vi "Main.vi"(8 "error in":errorcluster, 11 "Table in":refnum<class "Table.lvclass">) -> (0 "error out":errorcluster, 3 "Table out":refnum<class "Table.lvclass">)   [LabVIEW 2023, in "Table.lvclass"]
uses:
  Table.lvclass
  C:/Program Files (x86)/National Instruments/LabVIEW 2023/vi.lib/addons/_Workers/Library/Classes/Worker/Worker.lvclass
  <vilib>/addons/_Workers/Library/Classes/Worker/Worker.lvclass/Worker.ctl
  Philosopher/Initialization Data.ctl
  <vilib>/addons/_Workers/Library/Classes/Message Queue/Message Queue.lvclass
  Hungry.ctl
  Fork.ctl
  Philosopher/Philosopher.lvclass
  Table.lvclass/Table.ctl
  d0df4b09-6abd-41e7-b449-a85035083f06.vi
  <vilib>/addons/_Workers/Library/Classes/Message/Enqueue Message to Queue.vi
  <vilib>/addons/_Workers/Library/Classes/Worker/Worker.lvclass
  <vilib>/addons/_Workers/Library/Classes/Message/Message.lvclass
  C:/Program Files (x86)/National Instruments/LabVIEW 2023/vi.lib/addons/_Workers/Library/Classes/Workers Object/Workers Object.lvclass
  C:/Projects/DPP Workers/Workers/Table/Table.lvclass
panel:
  in  "The End":bool
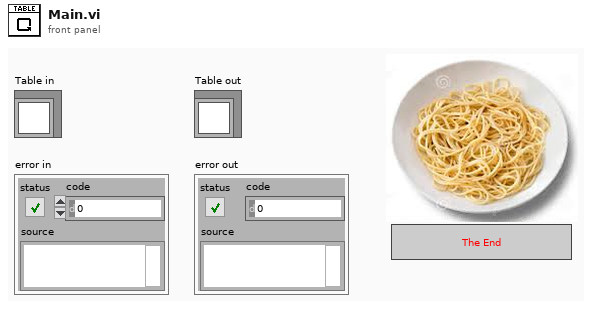
[diagram p1: front panel]
types:
  T1 = typedef "Philosopher.lvclass/Initialization Data.ctl" = cluster{"ID":i32, "MGQ Table":refnum<class "Message Queue.lvclass">}
  T2 = typedef "Table.lvclass/Hungry.ctl" = enum16{"NO", "YES"}
  T3 = typedef "Table.lvclass/Fork.ctl" = enum16{"FREE", "IN USE"}
  T4 = typedef "Workers.lvlib/Case Label.ctl" = string
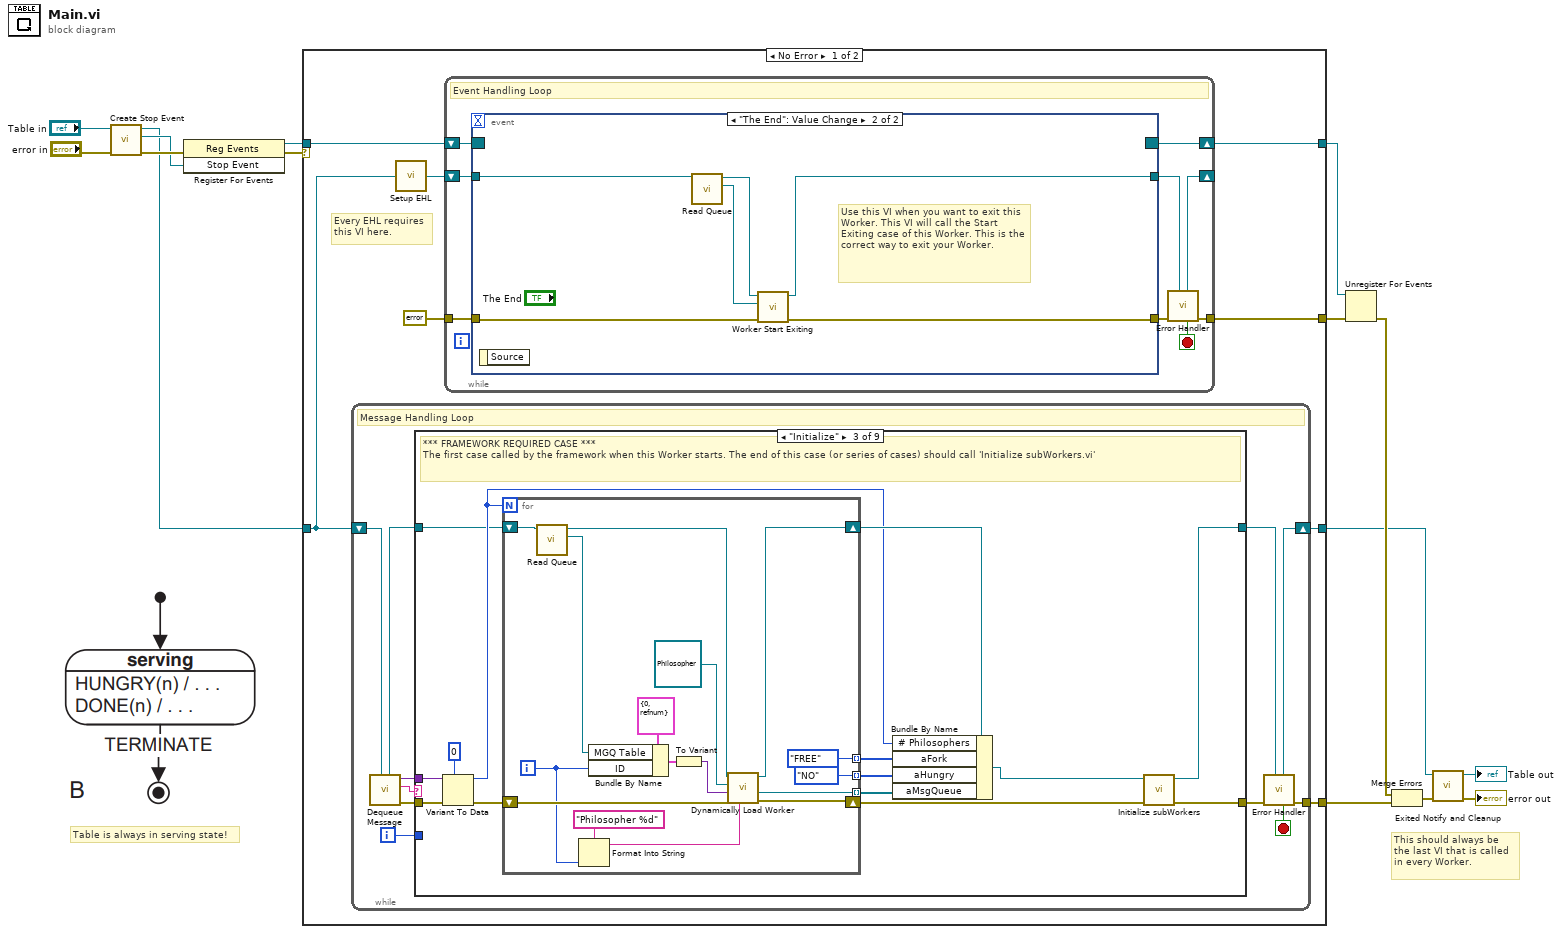
[diagram p0: block diagram]
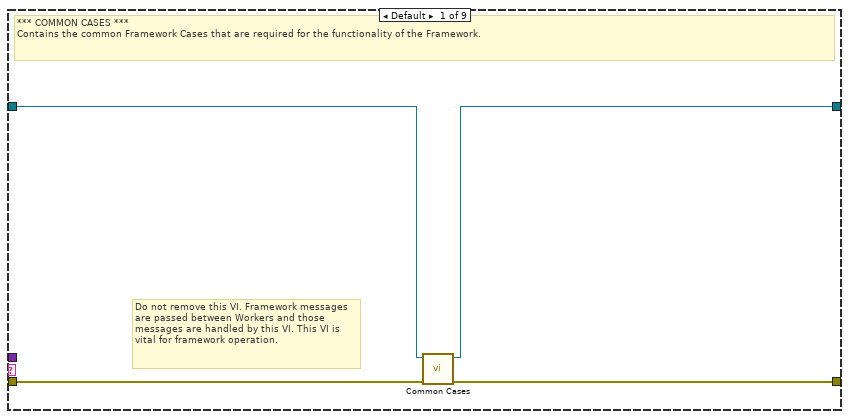
[diagram p2: hidden frame]
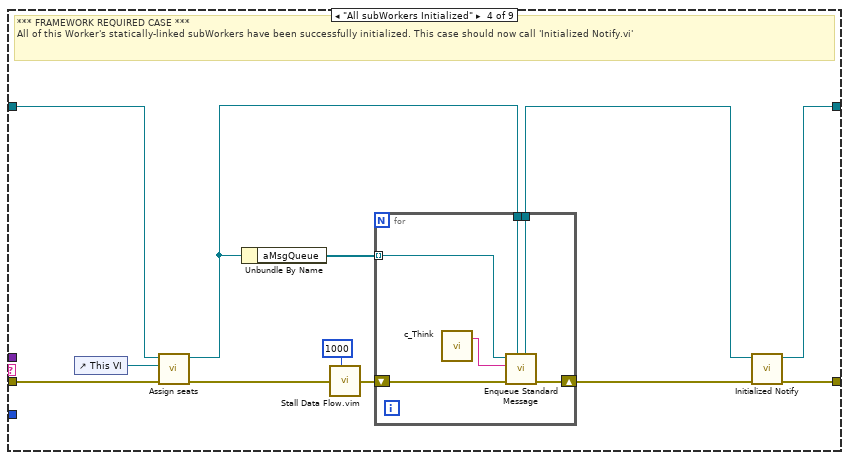
[diagram p4: hidden frame]
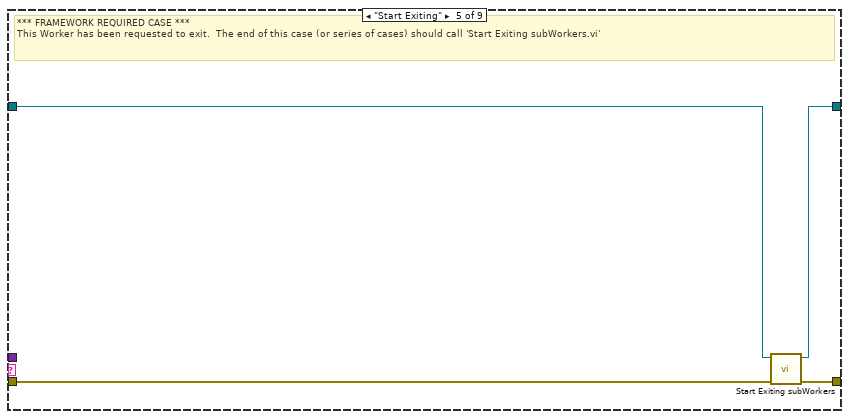
[diagram p5: hidden frame]
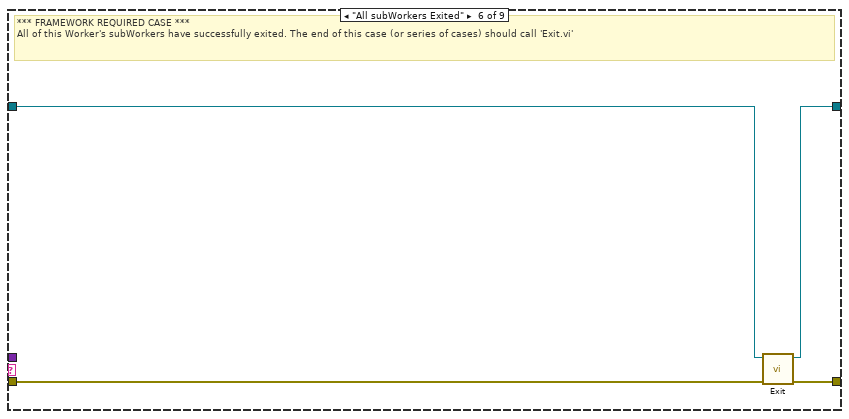
[diagram p6: hidden frame]
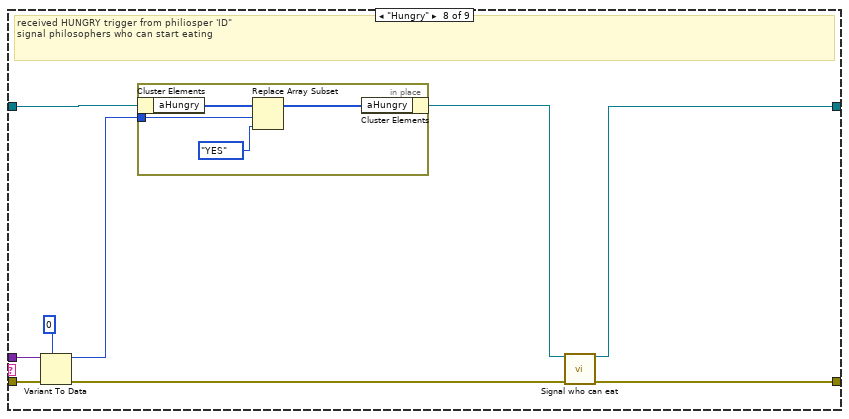
[diagram p8: hidden frame]
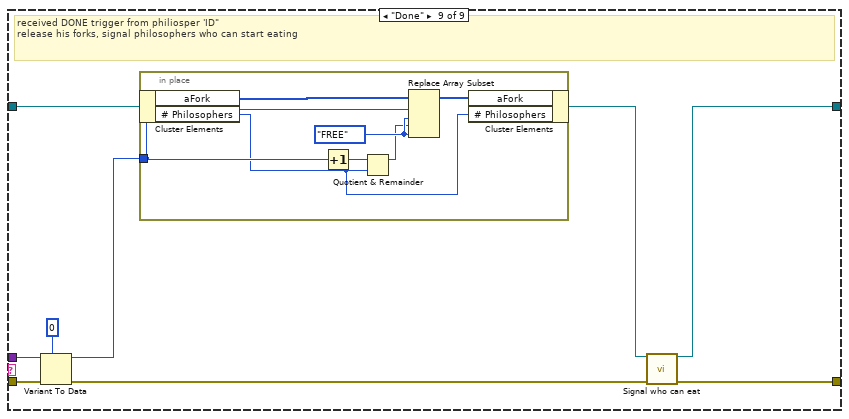
[diagram p9: hidden frame]
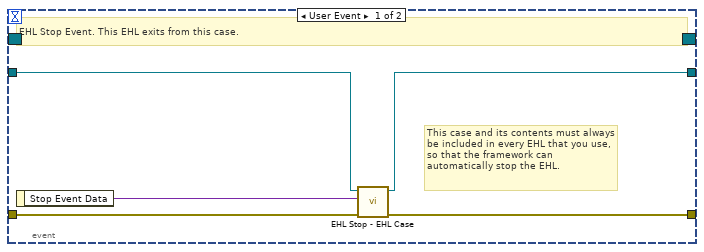
[diagram p10: hidden frame]
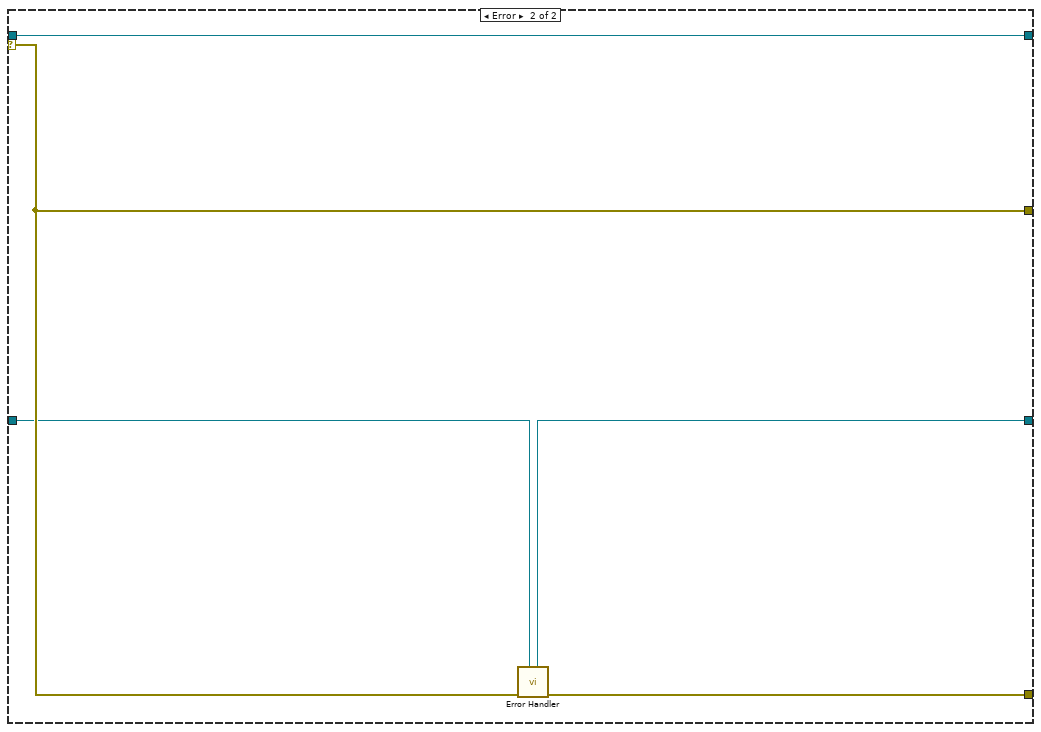
[diagram p11: hidden frame]
diagram:
  # "Table is always in serving state!"
  # "This should always be the last VI that is called in every Worker."
  n1 = call-dynamic "Create Stop Event.vi"("error in"="error in", "Worker"="Table in") -> ("error out"=w10:errorcluster, "Stop Event"=w7:refnum<user-event>, "Worker out"=w4:refnum<class "Table.lvclass">)  [unwired: 7 in]
  n2 = register-events(error in=w10, w7) -> (reference out=w9:refnum<event-registration>, error out=w2:errorcluster)  [unwired: 1 in]
  n3 = case shown="No Error" w2 {
    tunnel: w4 -> [w18 w149]
    tunnel: [w16 w150] -> w8
    tunnel: w9 -> [w23 w151]
    tunnel: [w20 w152] -> w14
    tunnel: [w22 w151] -> w13
    tunnel: [w17 w148] -> w11
    selector: w2 -> [_ w152]
    frame No Error {
      # "Every EHL requires\nthis VI here."
      n4 = while {
        shift-right: [w32] -> w17
        shift-left: w18 -> [w34]
        tunnel: [w33] -> w16
        i -> [w24]
        stop <- w25 stop-if-true
        # "Message Handling Loop"
        n5 = call-dynamic "Dequeue Message.vi"("Worker"=w34) -> ("error out"=w31:errorcluster, "Case out"=w26:string, "Data out"=w27:variant, "Worker out"=w29:refnum<class "Table.lvclass">)  [unwired: 6 in, 1 out]
        n6 = case "Worker MHL Case Structure (DO NOT CHANGE LABEL NAME)" shown="\"Initialize\"" w26 {
          tunnel: w31 -> [w38 w39 w52 w75 w89 w96 w97 w107 w120]
          tunnel: [w37 w39 w54 w79 w92 w95 w97 w102 w115] -> w30
          tunnel: w29 -> [w36 w40 w41 w73 w90 w94 w98 w101 w113]
          tunnel: [w35 w40 w53 w77 w91 w93 w98 w104 w117] -> w28
          tunnel: w27 -> [_ _ w51 _ _ _ _ w106 w119]
          tunnel: w24 -> [_ _ _ _ _ _ _ _ _]
          frame Default {
            # "Do not remove this VI. Framework messages are passed between Workers and those messages are handled by this VI. This VI is vital for framework operation."
            # "*** COMMON CASES ***\nContains the common Framework Cases that are required for the functionality of the Framework."
            n7 = call-dynamic "Common Cases.vi"("error in"=w38, "Worker in"=w36) -> ("error out"=w37:errorcluster, "Worker out"=w35:refnum<class "Table.lvclass">)  [unwired: 8 in]
          }
          frame "------ FRAMEWORK REQUIRED CASES ------" {
            # "Start of Framework Required Cases"
          }
          frame "Initialize" {
            # "*** FRAMEWORK REQUIRED CASE ***\nThe first case called by the framework when this Worker starts. The end of this case (or series of cases) should call 'Initialize subWorkers.vi'"
            n8 = Variant To Data(error in=w52, type=0 ("# Philosophers"), Variant=w51) -> (data=w44:i32, error out=w49:errorcluster)
            n9 = for {
              N: w44 -> [_]
              shift-right: [w69] -> w42
              shift-left: w49 -> [w70]
              shift-right: [w67] -> w48
              shift-left: w41 -> [w58]
              tunnel: [w63] -> w47 mode=indexing
              tunnel: [Fork."FREE" ("Fork")] -> w46 mode=indexing
              tunnel: [Hungry."NO" ("Hungry")] -> w45 mode=indexing
              i -> [w55]
              n10 = call <vilib>:"Read Queue.vi"("Worker"=w58) -> ("Message Queue out"=w56:refnum<class "Message Queue.lvclass">, "dup Worker out"=w57:refnum<class "Table.lvclass">)  [unwired: 9 in]
              n11 = Format Into String(format string="Philosopher %d", w55) -> (resulting string=w64:string)  [unwired: 2 in, 1 out]
              n12 = Bundle By Name(cluster=T1 {"ID"=0, "MGQ Table"=refnum} ("Initialization Data"), "MGQ Table"=w56, "ID"=w55) -> (w59:T1)
              n13 = To Variant(anything=w59) -> (Variant=w66:variant)
              n14 = call <vilib>:"Dynamically Load Worker.vi"("Worker Alias"=w64, "error in"=w70, "Initialization Data"=w66, "Worker to Dynamically Load"=refnum<class "Philosopher.lvclass"> refnum ("Philosopher.lvclass"), "Worker"=w57) -> ("error out"=w69:errorcluster, "Message Queue out"=w63:refnum<class "Message Queue.lvclass">, "dup Worker out"=w67:refnum<class "Table.lvclass">)  [unwired: 3 in, 1 out]
            }
            n15 = Bundle By Name(cluster=w48, "# Philosophers"=w44, "aFork"=w46, "aHungry"=w45, "aMsgQueue"=w47) -> (w43:refnum<class "Table.lvclass">)
            n16 = call-dynamic "Initialize subWorkers.vi"("error in"=w42, "Worker"=w43) -> ("error out"=w54:errorcluster, "dup Worker out"=w53:refnum<class "Table.lvclass">)  [unwired: 8 in]
          }
          frame "All subWorkers Initialized" {
            # "*** FRAMEWORK REQUIRED CASE ***\nAll of this Worker's statically-linked subWorkers have been successfully initialized. This case should now call 'Initialized Notify.vi'"
            n17 = control-ref of="This VI"() -> (w76:refnum<vi>)
            n18 = call "Assign seats.vi"("error in"=w75, "ref. Table"=w76, "Table in"=w73) -> ("error out"=w72:errorcluster, "Table out"=w74:refnum<class "Table.lvclass">)  [unwired: 7 in]
            n19 = Unbundle By Name(w74) -> ("aMsgQueue"=w82:refnum<class "Message Queue.lvclass">[])
            n20 = call "Stall Data Flow.vim"("value in"=w72, "milliseconds to wait"=u32 1000) -> ("value out"=w81:errorcluster)  [unwired: 1 out]
            n21 = for {
              tunnel: w82 -> [w88] mode=indexing
              shift-right: [w86] -> w71
              shift-left: w81 -> [w87]
              tunnel: w74 -> [w85]
              tunnel: [w84] -> w78
              n22 = call "c_Think.vi"() -> ("Case Label"=w83:T4)  [unwired: 1 in]
              n23 = call-poly <vilib>:"Enqueue Standard Message.vi"("Worker"=w85, "error in"=w87, "Case Label"=w83, "Message Queue"=w88) -> ("error out"=w86:errorcluster, "dup Worker out"=w84:refnum<class "Table.lvclass">)  [unwired: 5 in, 1 out]
            }
            n24 = call-dynamic "Initialized Notify.vi"("error in"=w71, "Worker"=w78) -> ("error out"=w79:errorcluster, "dup Worker out"=w77:refnum<class "Table.lvclass">)  [unwired: 8 in]
          }
          frame "Start Exiting" {
            # "*** FRAMEWORK REQUIRED CASE ***\nThis Worker has been requested to exit.  The end of this case (or series of cases) should call 'Start Exiting subWorkers.vi'"
            n25 = call-dynamic "Start Exiting subWorkers.vi"("error_in"=w89, "Worker"=w90) -> ("error out"=w92:errorcluster, "dup Worker out"=w91:refnum<class "Table.lvclass">)  [unwired: 8 in]
          }
          frame "All subWorkers Exited" {
            # "*** FRAMEWORK REQUIRED CASE ***\nAll of this Worker's subWorkers have successfully exited. The end of this case (or series of cases) should call 'Exit.vi'"
            n26 = call-dynamic "Exit.vi"("error_in"=w96, "Worker"=w94) -> ("error out"=w95:errorcluster, "dup Worker out"=w93:refnum<class "Table.lvclass">)  [unwired: 8 in]
          }
          frame "-----------------------------------------------" {
            # "End of Framework Required Cases"
          }
          frame "Hungry" {
            # "received HUNGRY trigger from philiosper 'ID\"\nsignal philosophers who can start eating"
            n27 = Variant To Data(error in=w107, type=0 ("index"), Variant=w106) -> (data=w100:i32, error out=w103:errorcluster)
            n28 = in-place "In Place Element Structure" {
              in-place-border: w100 -> [w108]
              n29 = in-place-cluster #1(w101) -> ("aHungry"=w111:T2[])
              n30 = Replace Array Subset(array=w111, new element=Hungry."YES" ("new element/subarray"), index=w108) -> (w110:T2[])
              n31 = in-place-cluster #1("aHungry"=w110) -> (w99:refnum<class "Table.lvclass">)
            }
            n32 = call "Signal who can eat.vi"("Table in"=w99, "error in"=w103) -> ("Table out"=w104:refnum<class "Table.lvclass">, "error out"=w102:errorcluster)  [unwired: 12 in]
          }
          frame "Done" {
            # "received DONE trigger from philiosper 'ID\"\nrelease his forks, signal philosophers who can start eating"
            n33 = Variant To Data(error in=w120, type=0 ("index"), Variant=w119) -> (data=w114:i32, error out=w116:errorcluster)
            n34 = in-place "In Place Element Structure" {
              in-place-border: w114 -> [w126]
              w125 = Fork."FREE" ("new element/subarray")
              n35 = in-place-cluster #2(w113) -> ("aFork"=w123:T3[], "# Philosophers"=w121:i32)
              n36 = Increment(x=w126) -> (x+1=w127:i32)
              n37 = Quotient & Remainder(x=w127, y=w121) -> (x-y*floor(x/y)=w124:i32)  [unwired: 1 out]
              n38 = Replace Array Subset(array=w123, new element #1=w125, index #1=w126, new element #2=w125, index #2=w124) -> (w122:T3[])
              n39 = in-place-cluster #2("aFork"=w122, "# Philosophers"=w121) -> (w112:refnum<class "Table.lvclass">)
            }
            n40 = call "Signal who can eat.vi"("Table in"=w112, "error in"=w116) -> ("Table out"=w117:refnum<class "Table.lvclass">, "error out"=w115:errorcluster)  [unwired: 12 in]
          }
        }
        n41 = call-dynamic "Error Handler.vi"("Worker"=w28, "error_in"=w30) -> ("error out"=w33:errorcluster, "Stop Loop"=w25:bool, "Worker out"=w32:refnum<class "Table.lvclass">)  [unwired: 7 in]
      }
      n42 = call-dynamic "Setup EHL.vi"("Worker"=w18) -> ("Worker out"=w19:refnum<class "Table.lvclass">)  [unwired: 14 in]
      n43 = while "Event Handling Loop" {
        shift-right: [w136] -> w22
        shift-left: w23 -> [w135]
        tunnel: [w131] -> w20
        tunnel: errorcluster {"status"=FALSE, "code"=0, "source"=""} ("error constant") -> [w133]
        shift-right: [w129] -> _
        shift-left: w19 -> [w134]
        stop <- w128 stop-if-true
        # "Event Handling Loop"
        n44 = event shown="[1] \"The End\": Value Change" {
          selector: w135 -> [_ _]
          dyn-events: [_ _] -> w136
          timeout: _ -> [_ _]
          tunnel: [w140 w144] -> w132
          tunnel: w133 -> [w141 w145]
          tunnel: w134 -> [w139 w143]
          tunnel: [w138 w142] -> w130
          event User Event {
            # "This case and its contents must always be included in every EHL that you use, so that the framework can automatically stop the EHL."
            # "EHL Stop Event. This EHL exits from this case."
            n45 = event-data() -> ("Stop Event Data"=w137:variant)  [unwired: 1 in]
            n46 = call <vilib>:"EHL Stop - EHL Case.vi"("error in"=w141, "Stop Event Data"=w137, "Worker"=w139) -> ("error out"=w140:errorcluster, "Worker out"=w138:refnum<class "Table.lvclass">)  [unwired: 7 in]
          }
          event "The End": Value Change {
            # "Use this VI when you want to exit this Worker. This VI will call the Start Exiting case of this Worker. This is the correct way to exit your Worker."
            n47 = event-data() -> ()  [unwired: 1 in, 1 out]
            n48 = call <vilib>:"Read Queue.vi"("Worker"=w143) -> ("Message Queue out"=w146:refnum<class "Message Queue.lvclass">, "dup Worker out"=w147:refnum<class "Table.lvclass">)  [unwired: 9 in]
            n49 = call-dynamic "Worker Start Exiting.vi"("error_in"=w145, "Message Queue"=w146, "Worker"=w147) -> ("error out"=w144:errorcluster, "dup Worker out"=w142:refnum<class "Table.lvclass">)  [unwired: 7 in]
          }
        }
        n50 = call-dynamic "Error Handler.vi"("Worker"=w130, "error_in"=w132) -> ("error out"=w131:errorcluster, "Stop Loop"=w128:bool, "Worker out"=w129:refnum<class "Table.lvclass">)  [unwired: 7 in]
      }
    }
    frame Error {
      n51 = call-dynamic "Error Handler.vi"("Worker"=w149, "error_in"=w152) -> ("error out"=w150:errorcluster, "Worker out"=w148:refnum<class "Table.lvclass">)  [unwired: 7 in, 1 out]
    }
  }
  n52 = Unregister For Events(event registration refnum=w13, error in=w14) -> (error out=w15:errorcluster)
  n53 = Merge Errors(w15, w8) -> (w12:errorcluster)
  n54 = call-dynamic "Exited Notify and Cleanup.vi"("error_in"=w12, "Worker"=w11) -> ("error out"=→"error out":errorcluster, "dup Worker out"=→"Table out":refnum<class "Table.lvclass">)  [unwired: 8 in]
